vi "Check Action.vi"(6 "HRS Time":dbl, 7 "Values In":dbl[](array[numeric]), 8 "error in (no error)":errorcluster, 11 "Valve in":refnum<class "LimitControl.lvclass">) -> (0 "error out":errorcluster, 2 "Actions":T1[](array[typedef]), 3 "Valve out":refnum<class "LimitControl.lvclass">, 5 "Values":dbl[](array[numeric]))   [LabVIEW 2020, in "VolatusControl.lvlib" / "LimitControl.lvclass"]
uses:
  LimitControl.lvclass
  Control Action.ctl
  LimitControl.lvclass/LimitControl.ctl
  lv-vecto/Vecto/Vecto.lvlib
  Volatus/MessageQ/MessageQ.lvclass
  VolatusControl.lvlib
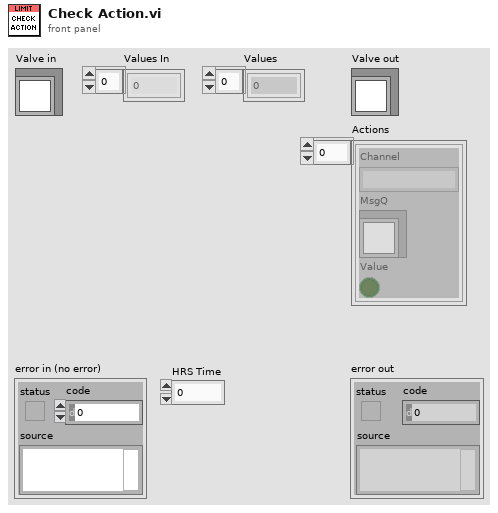
[diagram p1: front panel]
types:
  T1 = typedef "VolatusControl.lvlib/Control Action.ctl" = cluster{"Channel":string, "MsgQ":refnum<class "MessageQ.lvclass">, "Value":bool}
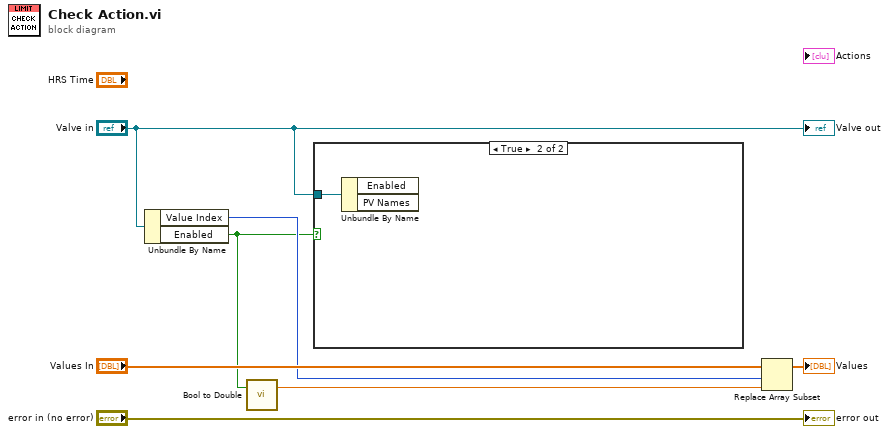
[diagram p0: block diagram]
diagram:
  n1 = Unbundle By Name("Valve in") -> ("Value Index"=w4:i32, "Enabled"=w2:bool)
  n2 = call "Bool to Double.vi"("Bool"=w2) -> ("Double"=w3:dbl)  [unwired: 2 in]
  n3 = case shown="True" w2 {
    tunnel: "Valve in" -> [_ w8]
    frame False {
    }
    frame True {
      n4 = Unbundle By Name(w8) -> ()  [unwired: 2 out]
    }
  }
  n5 = Replace Array Subset(array="Values In", new element=w3, index=w4) -> (→"Values":dbl[])
  "error out" <- "error in (no error)"
  "Valve out" <- "Valve in"
